vi "Current VIs Path.vi"(8 "error in (no error)":errorcluster) -> (0 "error out":errorcluster, 3 "Current VI's Path":path)   [LabVIEW 2010, in "Core SubVIs.lvlib"]
uses:
  Core SubVIs.lvlib
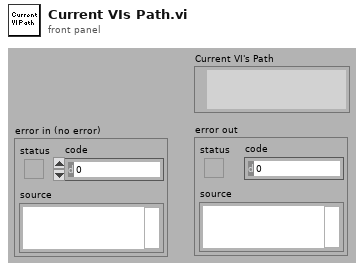
[diagram p1: front panel]
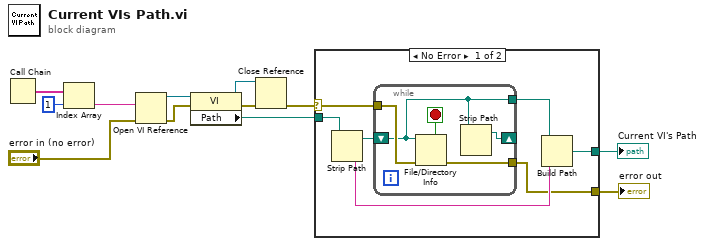
[diagram p0: block diagram]
diagram:
  n1 = Call Chain() -> (call chain=w12:string[])
  n2 = Index Array(array=w12, index=1) -> (element=w10:string)
  n3 = Open VI Reference(vi path=w10, error in (no error)="error in (no error)") -> (vi reference=w8:refnum<vi>, error out=w7:errorcluster)  [unwired: 4 out]
  n4 = property class="VI"(reference=w8, error in=w7) -> (reference out=w4:refnum<vi>, error out=w3:errorcluster, "Path"=w6:path)
  n5 = Close Reference(reference=w4, error in (no error)=w3) -> (error out=w1:errorcluster)
  n6 = case shown="No Error" w1 {
    selector: w1 -> [w14 w26]
    tunnel: w6 -> [w19 w25]
    tunnel: [w16 w25] -> w5
    tunnel: [w15 w26] -> w2
    frame No Error {
      n7 = Strip Path(path=w19) -> (stripped path=w13:path, name=w17:string)
      n8 = while {
        tunnel: w14 -> [w23]
        tunnel: [w21] -> w18
        tunnel: [w22] -> w15
        shift-right: [w20] -> _
        shift-left: w13 -> [w21]
        stop <- w24 stop-if-true
        n9 = File/Directory Info(path=w21, error in=w23) -> (directory=w24:bool, error out=w22:errorcluster)  [unwired: 5 out]
        n10 = Strip Path(path=w21) -> (stripped path=w20:path)  [unwired: 1 out]
      }
      n11 = Build Path(base path=w18, name or relative path=w17) -> (appended path=w16:path)
    }
    frame Error {
    }
  }
  "Current VI's Path" <- w5
  "error out" <- w2
